vi "GetFirstProcessModule.vi"   [LabVIEW 2017, in "FileFlow.lvlib"]
doc: "Sends an in-memory TDMS file to the first process in the Fileflow Script via a Qbus message. The first process operates on the file and then transfers it to the next process."
uses:
  <vilib>/addons/InsightCM/Devices/Shared/Common/FileFlow/FileFlow.lvlib
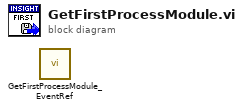
[diagram p0: block diagram]
diagram:
  n1 = call <vilib>:"GetFirstProcessModule_EventRef.vi"() -> ()  [unwired: 10 in, 2 out]
